vi "3010_2CAM.VI"() -> ()   [LabVIEW 2015]
uses:
  board.vis/Globals.vi
  <vilib>/Analysis/NI_AALBase.lvlib
panel:
  out "Signalverlaufgraph Cam 2":u16[](graph)=[28, 28, 29, 29, 30, 30, 31, 31, 32, 32, 33, 33, 34, 34, 35, 35, 36, 36, 37, 37, 38, 38, 39, 39, 40, 40, 41, 41, 42, 42, 43, 43, 44, 44, 45, 45, 46, 46, 47, 47, 48, 48, 49, 49, 50, 50, 51, 51, 52, 52, 53, 53, 54, 54, 55, 55, 56, 56, 57, 57, 58, 58, 59, 59, 60, 60, 61, 61, 62, 62, 63, 63, 64, 64, 65, 65, 66, 66, 67, 67, 68, 68, 69, 69, 70, 70, 71, 71, 72, 72, 73, 73, 74, 74, 75, 75, 76, 76, 77, 77, 78, 78, 79, 79, 80, 80, 81, 81, 82, 82, 83, 83, 84, 84, 85, 85, 86, 86, 87, 87, 88, 88, 89, 89, 90, 90, 91, 91, 92, 92, 93, 93, 94, 94, 95, 95, 96, 96, 97, 97, 98, 98, 99, 99, 100, 100, 101, 101, 102, 102, 103, 103, 104, 104, 105, 105, 106, 106, 107, 107, 108, 108, 109, 109, 110, 110, 111, 111, 112, 112, 113, 113, 114, 114, 115, 115, 116, 116, 117, 117, 118, 118, 119, 119, 120, 120, 121, 121, 122, 122, 123, 123, 124, 124, 125, 125, 126, 126, 127, 127, 128, 128, 129, 129, 130, 130, 131, 131, 132, 132, 133, 133, 134, 134, 135, 135, 136, 136, 137, 137, 138, 138, 139, 139, 140, 140, 141, 141, 142, 142, 143, 143, 144, 144, 145, 145, 146, 146, 147, 147, 148, 148, 149, 149, 150, 150, 151, 151, 152, 152, 153, 153, 154, 154, 155, 155, 156, 156, 157, 157, 158, 158, 159, 159, 160, 160, 161, 161, 162, 162, 163, 163, 164, 164, 165, 165, 166, 166, 167, 167, 168, 168, 169, 169, 170, 170, 171, 171, 172, 172, 173, 173, 174, 174, 175, 175, 176, 176, 177, 177, 178, 178, 179, 179, 180, 180, 181, 181, 182, 182, 183, 183, 184, 184, 185, 185, 186, 186, 187, 187, 188, 188, 189, 189, 190, 190, 191, 191, 192, 192, 193, 193, 194, 194, 195, 195, 196, 196, 197, 197, 198, 198, 199, 199, 200, 200, 201, 201, 202, 202, 203, 203, 204, 204, 205, 205, 206, 206, 207, 207, 208, 208, 209, 209, 210, 210, 211, 211, 212, 212, 213, 213, 214, 214, 215, 215, 216, 216, 217, 217, 218, 218, 219, 219, 220, 220, 221, 221, 222, 222, 223, 223, 224, 224, 225, 225, 226, 226, 227, 227, 228, 228, 229, 229, 230, 230, 231, 231, 232, 232, 233, 233, 234, 234, 235, 235, 236, 236, 237, 237, 238, 238, 239, 239, 240, 240, 241, 241, 242, 242, 243, 243, 244, 244, 245, 245, 246, 246, 247, 247, 248, 248, 249, 249, 250, 250, 251, 251, 252, 252, 253, 253, 254, 254, 255, 255, 256, 256, 257, 257, 258, 258, 259, 259, 260, 260, 261, 261, 262, 262, 263, 263, 264, 264, 265, 265, 266, 266, 267, 267, 268, 268, 269, 269, 270, 270, 271, 271, 272, 272, 273, 273, 274, 274, 275, 275, 276, 276, 277, 277, 278, 278, 279, 279, 280, 280, 281, 281, 282, 282, 283, 283, 284, 284, 285, 285, 286, 286, 287, 287, 288, 288, 289, 289, 290, 290, 291, 291, 292, 292, 293, 293, 294, 294, 295, 295, 296, 296, 297, 297, 298, 298, 299, 299, 300, 300, 301, 301, 302, 302, 303, 303, 304, 304, 305, 305, 306, 306, 307, 307, 308, 308, 309, 309, 310, 310, 311, 311, 312, 312, 313, 313, 314, 314, 315, 315, 316, 316, 317, 317, 318, 318, 319, 319, 320, 320, 321, 321, 322, 322, 323, 323, 324, 324, 325, 325, 326, 326, 327, 327, 328, 328, 329, 329, 330, 330, 331, 331, 332, 332, 333, 333, 334, 334, 335, 335, 336, 336, 337, 337, 338, 338, 339, 339, 340, 340, 341, 341, 342, 342, 343, 343, 344, 344, 345, 345, 346, 346, 347, 347, 348, 348, 349, 349, 350, 350, 351, 351, 352, 352, 353, 353, 354, 354, 355, 355, 356, 356, 357, 357, 358, 358, 359, 359, 360, 360, 361, 361, 362, 362, 363, 363, 364, 364, 365, 365, 366, 366, 367, 367, 368, 368, 369, 369, 370, 370, 371, 371, 372, 372, 373, 373, 374, 374, 375, 375, 376, 376, 377, 377, 378, 378, 379, 379, 380, 380, 381, 381, 382, 382, 383, 383, 384, 384, 385, 385, 386, 386, 387, 387, 388, 388, 389, 389, 390, 390, 391, 391, 392, 392, 393, 393, 394, 394, 395, 395, 396, 396, 397, 397, 398, 398, 399, 399, 400, 400, 401, 401, 402, 402, 403, 403, 404, 404, 405, 405, 406, 406, 407, 407, 408, 408, 409, 409, 410, 410, 411, 411, 412, 412, 413, 413, 414, 414, 415, 415, 416, 416, 417, 417, 418, 418, 419, 419, 420, 420, 421, 421, 422, 422, 423, 423, 424, 424, 425, 425, 426, 426, 427, 427, 428, 428, 429, 429, 430, 430, 431, 431, 432, 432, 433, 433, 434, 434, 435, 435, 436, 436, 437, 437, 438, 438, 439, 439, 440, 440, 441, 441, 442, 442, 443, 443, 444, 444, 445, 445, 446, 446, 447, 447, 448, 448, 449, 449, 450, 450, 451, 451, 452, 452, 453, 453, 454, 454, 455, 455, 456, 456, 457, 457, 458, 458, 459, 459, 460, 460, 461, 461, 462, 462, 463, 463, 464, 464, 465, 465, 466, 466, 467, 467, 468, 468, 469, 469, 470, 470, 471, 471, 472, 472, 473, 473, 474, 474, 475, 475, 476, 476, 477, 477, 478, 478, 479, 479, 480, 480, 481, 481, 482, 482, 483, 483, 484, 484, 485, 485, 486, 486, 487, 487, 488, 488, 489, 489, 490, 490, 491, 491, 492, 492, 493, 493, 494, 494, 495, 495, 496, 496, 497, 497, 498, 498, 499, 499, 500, 500, 501, 501, 502, 502, 503, 503, 504, 504, 505, 505, 506, 506, 507, 507, 508, 508, 509, 509, 510, 510, 511, 511, 512, 512, 513, 513, 514, 514, 515, 515, 516, 516, 517, 517, 518, 518, 519, 519, 520, 520, 521, 521, 522, 522, 523, 523, 524, 524, 525, 525, 526, 526, 527, 527, 528, 528, 529, 529, 530, 530, 531, 531, 532, 532, 533, 533, 534, 534, 535, 535, 536, 536, 537, 537, 538, 538, 539, 539, 540, 540, 541, 541, 542, 542, 543, 543, 544, 544, 544, 544, 544, 544, 544, 544, 544, 544, 544, 544, 544, 544, 544, 544, 544, 544, 544, 544, 544, 544, 544, 544, 544, 544, 544, 544, 544, 544, 544, 544, 544, 544, 544, 544, 544, 544, 544, 544, 544, 544, 544, 544, 544, 544, 544, 544, 544, 544, 544, 544, 544, 544, 544, 544]
  in  "extTrig":bool
  in  "ext. trig. slope":enum32{"1", "2", "3"}(radio)
  out "tRMS":dbl=8.272957184592048 format="%0#.1f"
  out "mean":dbl=3064.5285285285286 format="%#_4f"
  in  "rms_pixel":u16=100
  in  "is FFT":bool=TRUE
  in  "IR gain":bool
  in  "continuous":bool
  out "curr.block":u8=10
  out "Measure ON":bool
  in  "Board select\n1: board 1\n2: board 2\n3: both boards":u8=3
  in  "no.of blocks (nob)\npress enter":u32=1
  in  "block":u32(slide)=1 max=10 scale=0.9..1.0
  out "Signalverlaufgraph Board 2":u16[](graph)=[0, 0, 543, 543, 0, 1, 0, 0, 2, 2, 3, 3, 4, 4, 5, 5, 6, 6, 7, 7, 8, 8, 9, 9, 10, 10, 11, 11, 12, 12, 13, 13, 14, 14, 15, 15, 16, 16, 17, 17, 18, 18, 19, 19, 20, 20, 21, 21, 22, 22, 23, 23, 24, 24, 25, 25, 26, 26, 27, 27, 28, 28, 29, 29, 30, 30, 31, 31, 32, 32, 33, 33, 34, 34, 35, 35, 36, 36, 37, 37, 38, 38, 39, 39, 40, 40, 41, 41, 42, 42, 43, 43, 44, 44, 45, 45, 46, 46, 47, 47, 48, 48, 49, 49, 50, 50, 51, 51, 52, 52, 53, 53, 54, 54, 55, 55, 56, 56, 57, 57, 58, 58, 59, 59, 60, 60, 61, 61, 62, 62, 63, 63, 64, 64, 65, 65, 66, 66, 67, 67, 68, 68, 69, 69, 70, 70, 71, 71, 72, 72, 73, 73, 74, 74, 75, 75, 76, 76, 77, 77, 78, 78, 79, 79, 80, 80, 81, 81, 82, 82, 83, 83, 84, 84, 85, 85, 86, 86, 87, 87, 88, 88, 89, 89, 90, 90, 91, 91, 92, 92, 93, 93, 94, 94, 95, 95, 96, 96, 97, 97, 98, 98, 99, 99, 100, 100, 101, 101, 102, 102, 103, 103, 104, 104, 105, 105, 106, 106, 107, 107, 108, 108, 109, 109, 110, 110, 111, 111, 112, 112, 113, 113, 114, 114, 115, 115, 116, 116, 117, 117, 118, 118, 119, 119, 120, 120, 121, 121, 122, 122, 123, 123, 124, 124, 125, 125, 126, 126, 127, 127, 128, 128, 129, 129, 130, 130, 131, 131, 132, 132, 133, 133, 134, 134, 135, 135, 136, 136, 137, 137, 138, 138, 139, 139, 140, 140, 141, 141, 142, 142, 143, 143, 144, 144, 145, 145, 146, 146, 147, 147, 148, 148, 149, 149, 150, 150, 151, 151, 152, 152, 153, 153, 154, 154, 155, 155, 156, 156, 157, 157, 158, 158, 159, 159, 160, 160, 161, 161, 162, 162, 163, 163, 164, 164, 165, 165, 166, 166, 167, 167, 168, 168, 169, 169, 170, 170, 171, 171, 172, 172, 173, 173, 174, 174, 175, 175, 176, 176, 177, 177, 178, 178, 179, 179, 180, 180, 181, 181, 182, 182, 183, 183, 184, 184, 185, 185, 186, 186, 187, 187, 188, 188, 189, 189, 190, 190, 191, 191, 192, 192, 193, 193, 194, 194, 195, 195, 196, 196, 197, 197, 198, 198, 199, 199, 200, 200, 201, 201, 202, 202, 203, 203, 204, 204, 205, 205, 206, 206, 207, 207, 208, 208, 209, 209, 210, 210, 211, 211, 212, 212, 213, 213, 214, 214, 215, 215, 216, 216, 217, 217, 218, 218, 219, 219, 220, 220, 221, 221, 222, 222, 223, 223, 224, 224, 225, 225, 226, 226, 227, 227, 228, 228, 229, 229, 230, 230, 231, 231, 232, 232, 233, 233, 234, 234, 235, 235, 236, 236, 237, 237, 238, 238, 239, 239, 240, 240, 241, 241, 242, 242, 243, 243, 244, 244, 245, 245, 246, 246, 247, 247, 248, 248, 249, 249, 250, 250, 251, 251, 252, 252, 253, 253, 254, 254, 255, 255, 256, 256, 257, 257, 258, 258, 259, 259, 260, 260, 261, 261, 262, 262, 263, 263, 264, 264, 265, 265, 266, 266, 267, 267, 268, 268, 269, 269, 270, 270, 271, 271, 272, 272, 273, 273, 274, 274, 275, 275, 276, 276, 277, 277, 278, 278, 279, 279, 280, 280, 281, 281, 282, 282, 283, 283, 284, 284, 285, 285, 286, 286, 287, 287, 288, 288, 289, 289, 290, 290, 291, 291, 292, 292, 293, 293, 294, 294, 295, 295, 296, 296, 297, 297, 298, 298, 299, 299, 300, 300, 301, 301, 302, 302, 303, 303, 304, 304, 305, 305, 306, 306, 307, 307, 308, 308, 309, 309, 310, 310, 311, 311, 312, 312, 313, 313, 314, 314, 315, 315, 316, 316, 317, 317, 318, 318, 319, 319, 320, 320, 321, 321, 322, 322, 323, 323, 324, 324, 325, 325, 326, 326, 327, 327, 328, 328, 329, 329, 330, 330, 331, 331, 332, 332, 333, 333, 334, 334, 335, 335, 336, 336, 337, 337, 338, 338, 339, 339, 340, 340, 341, 341, 342, 342, 343, 343, 344, 344, 345, 345, 346, 346, 347, 347, 348, 348, 349, 349, 350, 350, 351, 351, 352, 352, 353, 353, 354, 354, 355, 355, 356, 356, 357, 357, 358, 358, 359, 359, 360, 360, 361, 361, 362, 362, 363, 363, 364, 364, 365, 365, 366, 366, 367, 367, 368, 368, 369, 369, 370, 370, 371, 371, 372, 372, 373, 373, 374, 374, 375, 375, 376, 376, 377, 377, 378, 378, 379, 379, 380, 380, 381, 381, 382, 382, 383, 383, 384, 384, 385, 385, 386, 386, 387, 387, 388, 388, 389, 389, 390, 390, 391, 391, 392, 392, 393, 393, 394, 394, 395, 395, 396, 396, 397, 397, 398, 398, 399, 399, 400, 400, 401, 401, 402, 402, 403, 403, 404, 404, 405, 405, 406, 406, 407, 407, 408, 408, 409, 409, 410, 410, 411, 411, 412, 412, 413, 413, 414, 414, 415, 415, 416, 416, 417, 417, 418, 418, 419, 419, 420, 420, 421, 421, 422, 422, 423, 423, 424, 424, 425, 425, 426, 426, 427, 427, 428, 428, 429, 429, 430, 430, 431, 431, 432, 432, 433, 433, 434, 434, 435, 435, 436, 436, 437, 437, 438, 438, 439, 439, 440, 440, 441, 441, 442, 442, 443, 443, 444, 444, 445, 445, 446, 446, 447, 447, 448, 448, 449, 449, 450, 450, 451, 451, 452, 452, 453, 453, 454, 454, 455, 455, 456, 456, 457, 457, 458, 458, 459, 459, 460, 460, 461, 461, 462, 462, 463, 463, 464, 464, 465, 465, 466, 466, 467, 467, 468, 468, 469, 469, 470, 470, 471, 471, 472, 472, 473, 473, 474, 474, 475, 475, 476, 476, 477, 477, 478, 478, 479, 479, 480, 480, 481, 481, 482, 482, 483, 483, 484, 484, 485, 485, 486, 486, 487, 487, 488, 488, 489, 489, 490, 490, 491, 491, 492, 492, 493, 493, 494, 494, 495, 495, 496, 496, 497, 497, 498, 498, 499, 499, 500, 500, 501, 501, 502, 502, 503, 503, 504, 504, 505, 505, 506, 506, 507, 507, 508, 508, 509, 509, 510, 510, 511, 511, 512, 512, 513, 513, 514, 514, 515, 515, 516, 516, 517, 517, 518, 518, 519, 519, 520, 520, 521, 521, 522, 522, 523, 523, 524, 524, 525, 525, 526, 526, 527, 527, 528, 528, 529, 529, 530, 530, 531, 531, 532, 532, 533, 533, 534, 534, 535, 535, 536, 536, 537, 537, 538, 538, 539, 539, 540, 540, 541, 541]
  out "Signalverlaufgraph":u16[](graph)=[544, 544, 545, 545, 49152, 1, 0, 148, 2, 2, 3, 3, 4, 4, 5, 5, 6, 6, 7, 7, 8, 8, 9, 9, 10, 10, 11, 11, 12, 12, 13, 13, 14, 14, 15, 15, 16, 16, 17, 17, 18, 18, 19, 19, 20, 20, 21, 21, 22, 22, 23, 23, 24, 24, 25, 25, 26, 26, 27, 27, 28, 28, 29, 29, 30, 30, 31, 31, 32, 32, 33, 33, 34, 34, 35, 35, 36, 36, 37, 37, 38, 38, 39, 39, 40, 40, 41, 41, 42, 42, 43, 43, 44, 44, 45, 45, 46, 46, 47, 47, 48, 48, 49, 49, 50, 50, 51, 51, 52, 52, 53, 53, 54, 54, 55, 55, 56, 56, 57, 57, 58, 58, 59, 59, 60, 60, 61, 61, 62, 62, 63, 63, 64, 64, 65, 65, 66, 66, 67, 67, 68, 68, 69, 69, 70, 70, 71, 71, 72, 72, 73, 73, 74, 74, 75, 75, 76, 76, 77, 77, 78, 78, 79, 79, 80, 80, 81, 81, 82, 82, 83, 83, 84, 84, 85, 85, 86, 86, 87, 87, 88, 88, 89, 89, 90, 90, 91, 91, 92, 92, 93, 93, 94, 94, 95, 95, 96, 96, 97, 97, 98, 98, 99, 99, 100, 100, 101, 101, 102, 102, 103, 103, 104, 104, 105, 105, 106, 106, 107, 107, 108, 108, 109, 109, 110, 110, 111, 111, 112, 112, 113, 113, 114, 114, 115, 115, 116, 116, 117, 117, 118, 118, 119, 119, 120, 120, 121, 121, 122, 122, 123, 123, 124, 124, 125, 125, 126, 126, 127, 127, 128, 128, 129, 129, 130, 130, 131, 131, 132, 132, 133, 133, 134, 134, 135, 135, 136, 136, 137, 137, 138, 138, 139, 139, 140, 140, 141, 141, 142, 142, 143, 143, 144, 144, 145, 145, 146, 146, 147, 147, 148, 148, 149, 149, 150, 150, 151, 151, 152, 152, 153, 153, 154, 154, 155, 155, 156, 156, 157, 157, 158, 158, 159, 159, 160, 160, 161, 161, 162, 162, 163, 163, 164, 164, 165, 165, 166, 166, 167, 167, 168, 168, 169, 169, 170, 170, 171, 171, 172, 172, 173, 173, 174, 174, 175, 175, 176, 176, 177, 177, 178, 178, 179, 179, 180, 180, 181, 181, 182, 182, 183, 183, 184, 184, 185, 185, 186, 186, 187, 187, 188, 188, 189, 189, 190, 190, 191, 191, 192, 192, 193, 193, 194, 194, 195, 195, 196, 196, 197, 197, 198, 198, 199, 199, 200, 200, 201, 201, 202, 202, 203, 203, 204, 204, 205, 205, 206, 206, 207, 207, 208, 208, 209, 209, 210, 210, 211, 211, 212, 212, 213, 213, 214, 214, 215, 215, 216, 216, 217, 217, 218, 218, 219, 219, 220, 220, 221, 221, 222, 222, 223, 223, 224, 224, 225, 225, 226, 226, 227, 227, 228, 228, 229, 229, 230, 230, 231, 231, 232, 232, 233, 233, 234, 234, 235, 235, 236, 236, 237, 237, 238, 238, 239, 239, 240, 240, 241, 241, 242, 242, 243, 243, 244, 244, 245, 245, 246, 246, 247, 247, 248, 248, 249, 249, 250, 250, 251, 251, 252, 252, 253, 253, 254, 254, 255, 255, 256, 256, 257, 257, 258, 258, 259, 259, 260, 260, 261, 261, 262, 262, 263, 263, 264, 264, 265, 265, 266, 266, 267, 267, 268, 268, 269, 269, 270, 270, 271, 271, 272, 272, 273, 273, 274, 274, 275, 275, 276, 276, 277, 277, 278, 278, 279, 279, 280, 280, 281, 281, 282, 282, 283, 283, 284, 284, 285, 285, 286, 286, 287, 287, 288, 288, 289, 289, 290, 290, 291, 291, 292, 292, 293, 293, 294, 294, 295, 295, 296, 296, 297, 297, 298, 298, 299, 299, 300, 300, 301, 301, 302, 302, 303, 303, 304, 304, 305, 305, 306, 306, 307, 307, 308, 308, 309, 309, 310, 310, 311, 311, 312, 312, 313, 313, 314, 314, 315, 315, 316, 316, 317, 317, 318, 318, 319, 319, 320, 320, 321, 321, 322, 322, 323, 323, 324, 324, 325, 325, 326, 326, 327, 327, 328, 328, 329, 329, 330, 330, 331, 331, 332, 332, 333, 333, 334, 334, 335, 335, 336, 336, 337, 337, 338, 338, 339, 339, 340, 340, 341, 341, 342, 342, 343, 343, 344, 344, 345, 345, 346, 346, 347, 347, 348, 348, 349, 349, 350, 350, 351, 351, 352, 352, 353, 353, 354, 354, 355, 355, 356, 356, 357, 357, 358, 358, 359, 359, 360, 360, 361, 361, 362, 362, 363, 363, 364, 364, 365, 365, 366, 366, 367, 367, 368, 368, 369, 369, 370, 370, 371, 371, 372, 372, 373, 373, 374, 374, 375, 375, 376, 376, 377, 377, 378, 378, 379, 379, 380, 380, 381, 381, 382, 382, 383, 383, 384, 384, 385, 385, 386, 386, 387, 387, 388, 388, 389, 389, 390, 390, 391, 391, 392, 392, 393, 393, 394, 394, 395, 395, 396, 396, 397, 397, 398, 398, 399, 399, 400, 400, 401, 401, 402, 402, 403, 403, 404, 404, 405, 405, 406, 406, 407, 407, 408, 408, 409, 409, 410, 410, 411, 411, 412, 412, 413, 413, 414, 414, 415, 415, 416, 416, 417, 417, 418, 418, 419, 419, 420, 420, 421, 421, 422, 422, 423, 423, 424, 424, 425, 425, 426, 426, 427, 427, 428, 428, 429, 429, 430, 430, 431, 431, 432, 432, 433, 433, 434, 434, 435, 435, 436, 436, 437, 437, 438, 438, 439, 439, 440, 440, 441, 441, 442, 442, 443, 443, 444, 444, 445, 445, 446, 446, 447, 447, 448, 448, 449, 449, 450, 450, 451, 451, 452, 452, 453, 453, 454, 454, 455, 455, 456, 456, 457, 457, 458, 458, 459, 459, 460, 460, 461, 461, 462, 462, 463, 463, 464, 464, 465, 465, 466, 466, 467, 467, 468, 468, 469, 469, 470, 470, 471, 471, 472, 472, 473, 473, 474, 474, 475, 475, 476, 476, 477, 477, 478, 478, 479, 479, 480, 480, 481, 481, 482, 482, 483, 483, 484, 484, 485, 485, 486, 486, 487, 487, 488, 488, 489, 489, 490, 490, 491, 491, 492, 492, 493, 493, 494, 494, 495, 495, 496, 496, 497, 497, 498, 498, 499, 499, 500, 500, 501, 501, 502, 502, 503, 503, 504, 504, 505, 505, 506, 506, 507, 507, 508, 508, 509, 509, 510, 510, 511, 511, 512, 512, 513, 513, 514, 514, 515, 515, 516, 516, 517, 517, 518, 518, 519, 519, 520, 520, 521, 521, 522, 522, 523, 523, 524, 524, 525, 525, 526, 526, 527, 527, 528, 528, 529, 529, 530, 530, 531, 531, 532, 532, 533, 533, 534, 534, 535, 535, 536, 536, 537, 537, 538, 538, 539, 539, 540, 540, 541, 541]
  out "boards recognised":u8=1
  in  "alloc mem":bool
  out "FREE \nRAM MB":dbl=14657.53515625
  out "BUILT-IN\nRAM MB":dbl=18096.171875
  out "SEC":dbl=1.0
  out "MB RAM":dbl=4.150390625
  in  "DAT in 10ns":u32
  in  "stop all":bool
  in  "start":bool
  in  "sample":u32(slide)=75 max=3000 scale=0.9..100.0
  in  "no.of samples (nos)":u32=100
  in  "exposuretime[ms]":dbl=1.0 format="%.3f"
  # "press Esc to stop measurement"
  # "exit here"
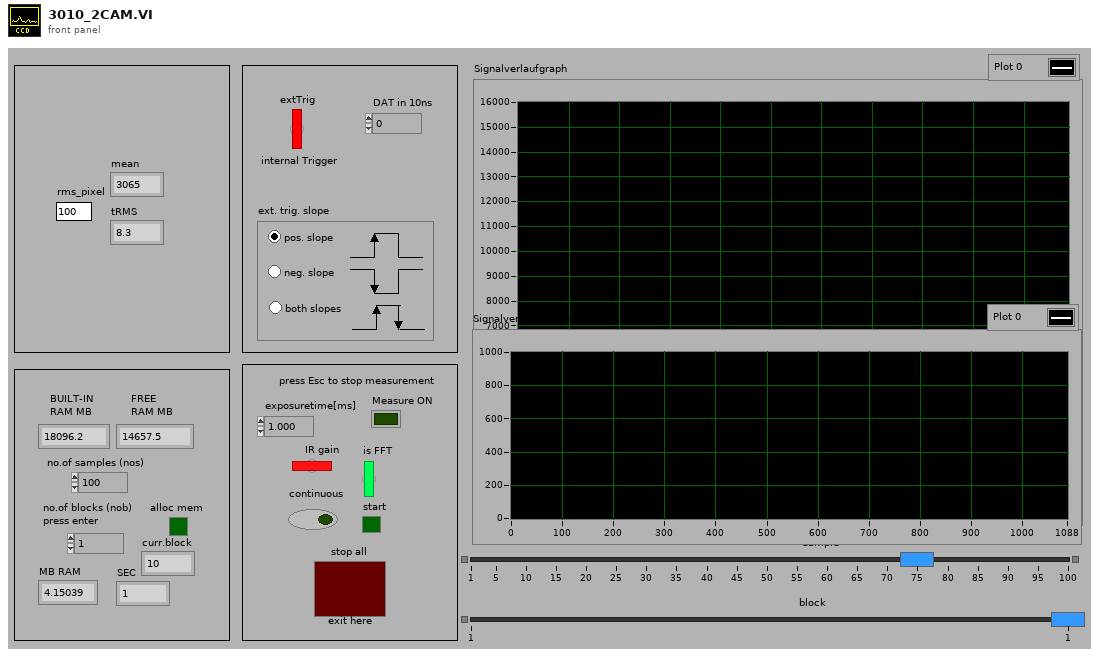
[diagram p1: front panel]
types:
  T1 = enum8{"Enabled", "Disabled", "Disabled and Grayed Out"}
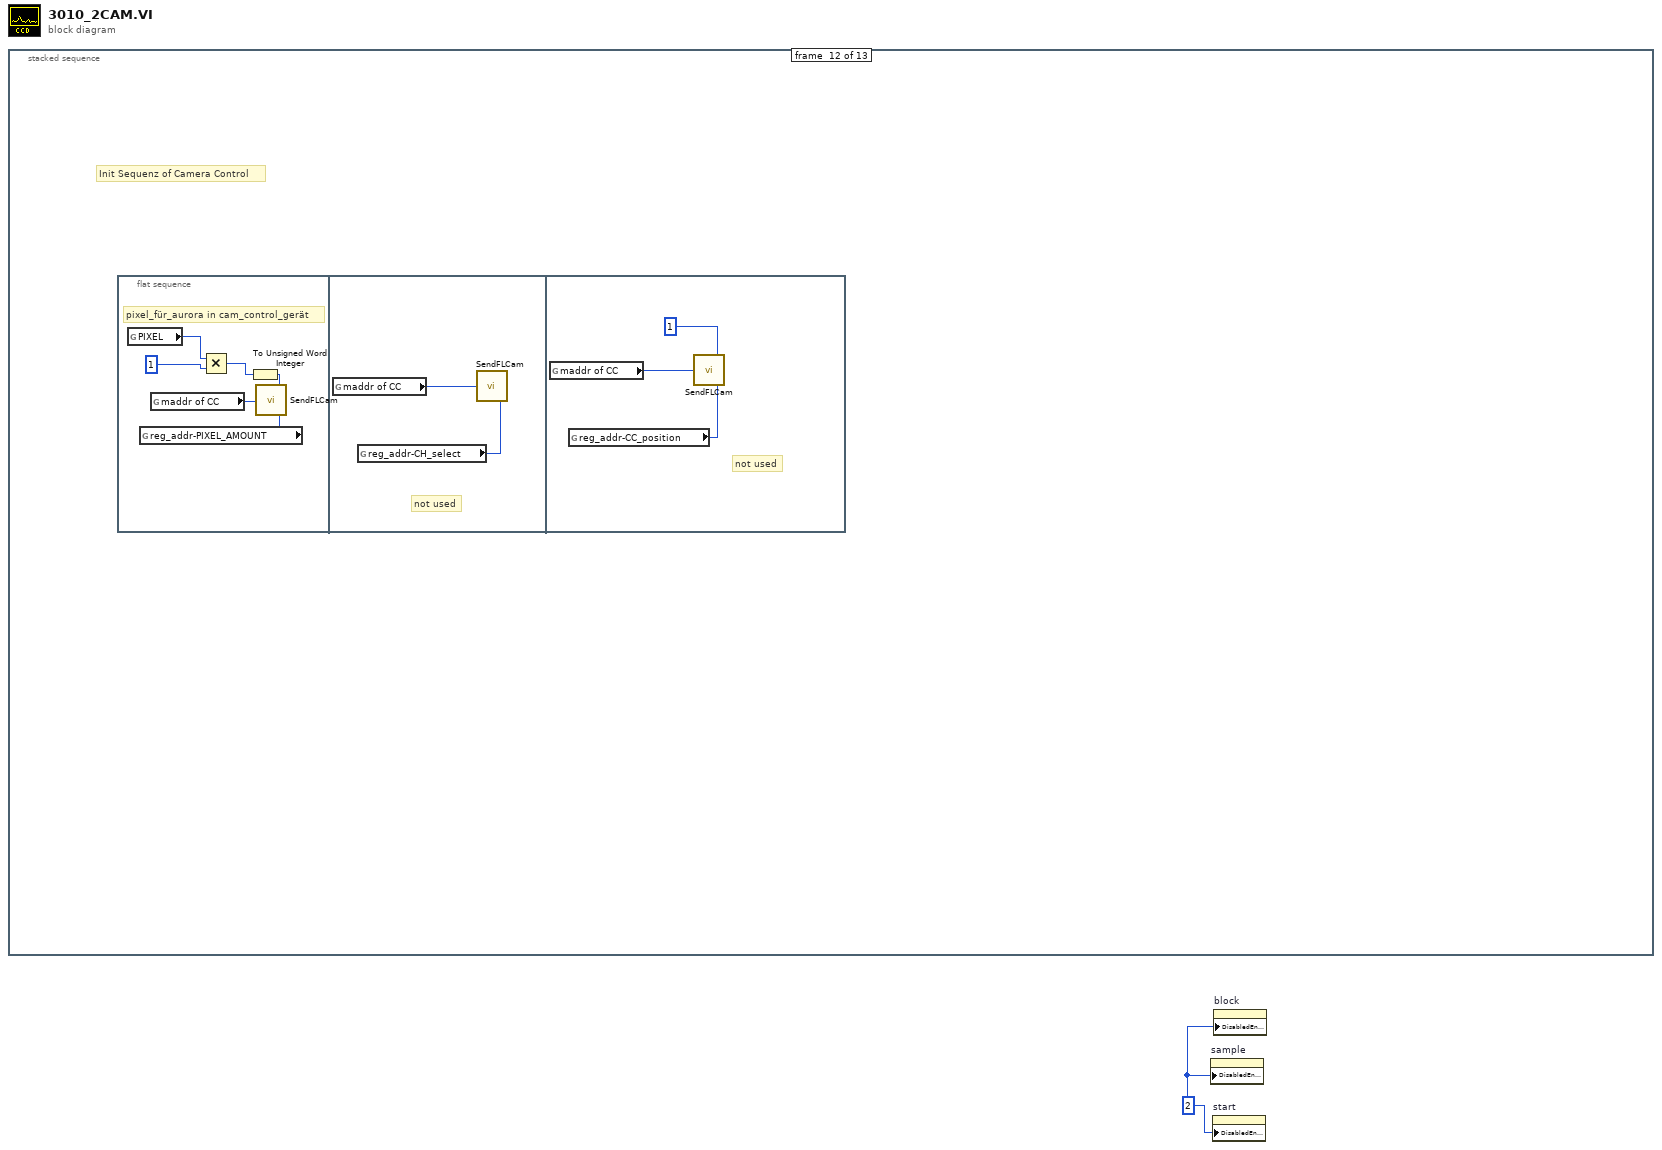
[diagram p0: block diagram]
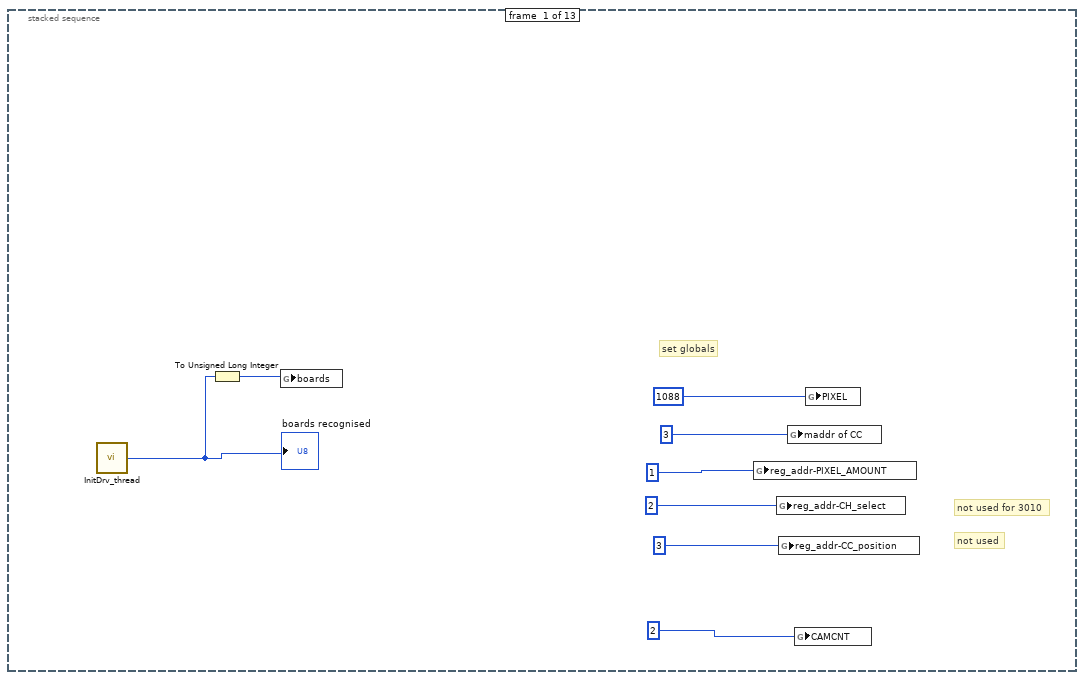
[diagram p2: hidden frame]
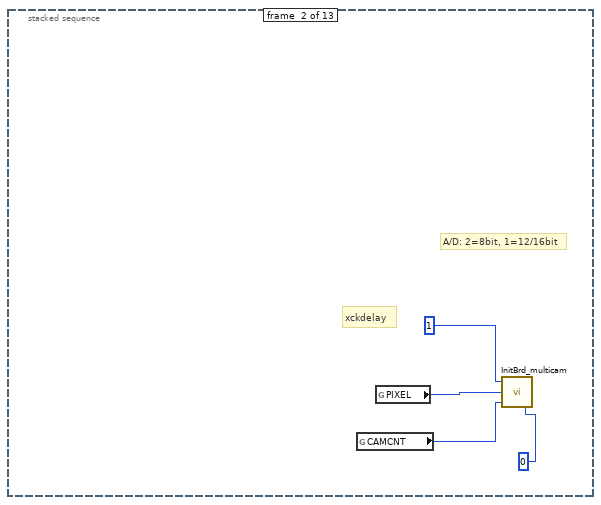
[diagram p3: hidden frame]
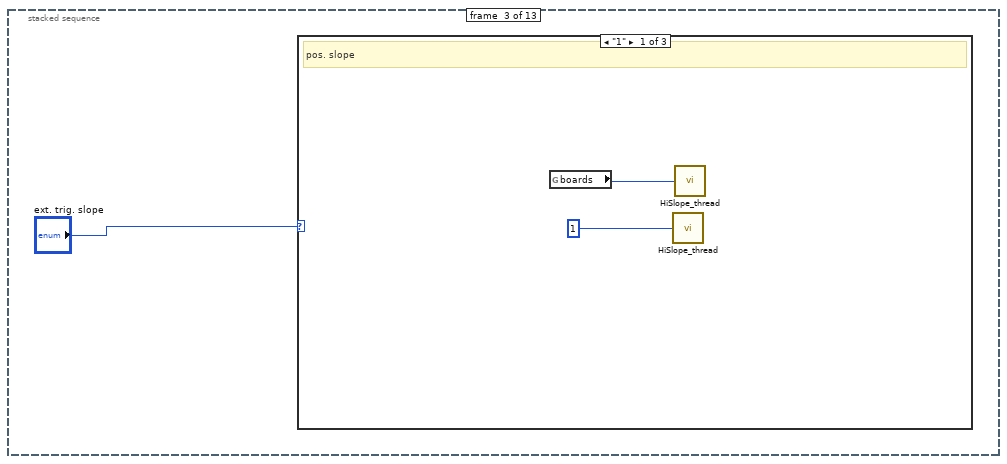
[diagram p4: hidden frame]
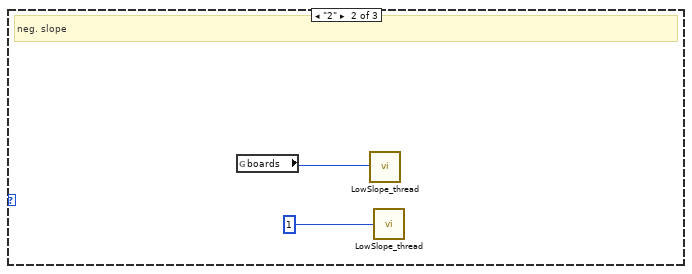
[diagram p5: hidden frame]
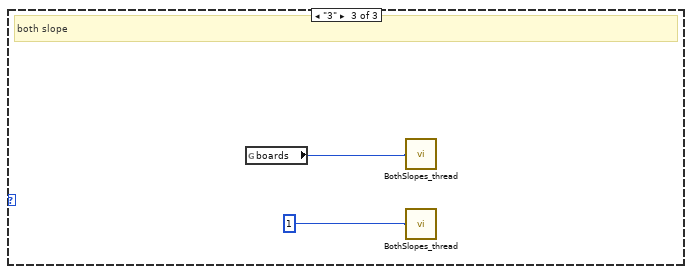
[diagram p6: hidden frame]
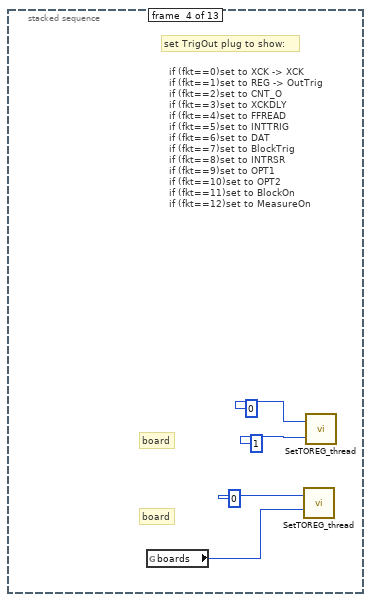
[diagram p7: hidden frame]
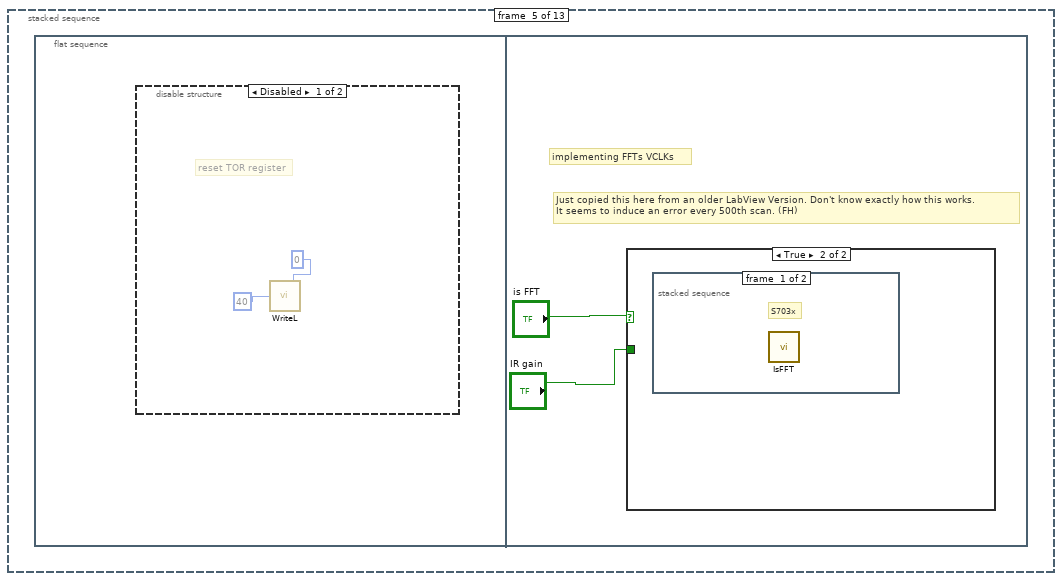
[diagram p8: hidden frame]
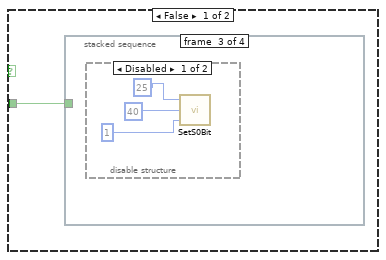
[diagram p10: hidden frame]
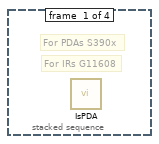
[diagram p11: hidden frame]
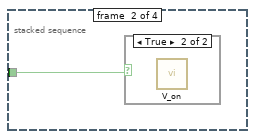
[diagram p12: hidden frame]
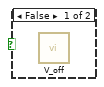
[diagram p13: hidden frame]
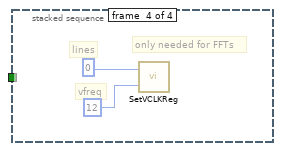
[diagram p15: hidden frame]
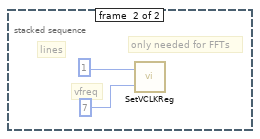
[diagram p16: hidden frame]
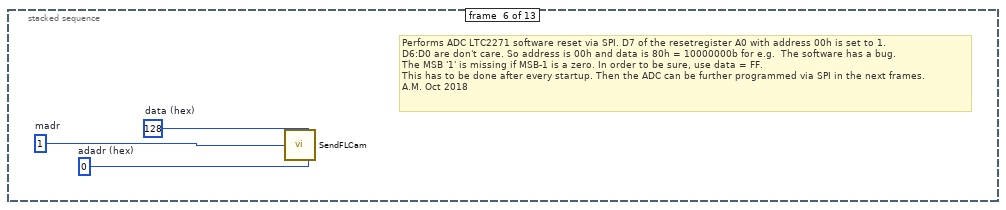
[diagram p17: hidden frame]
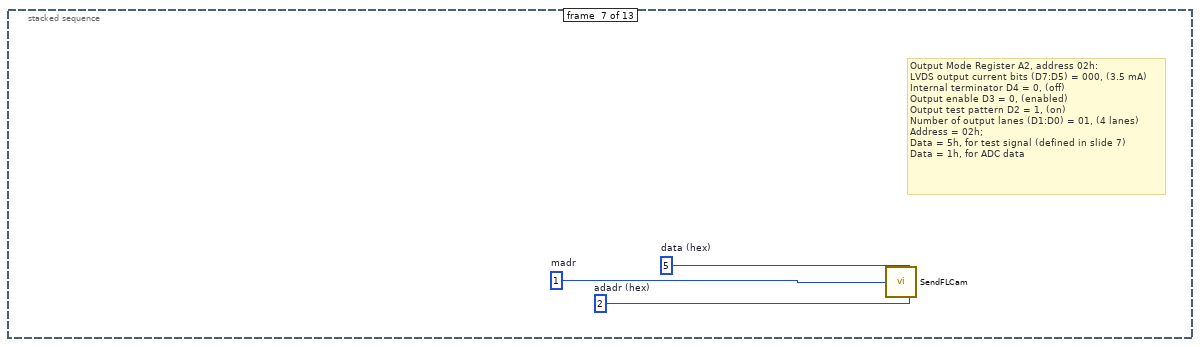
[diagram p18: hidden frame]
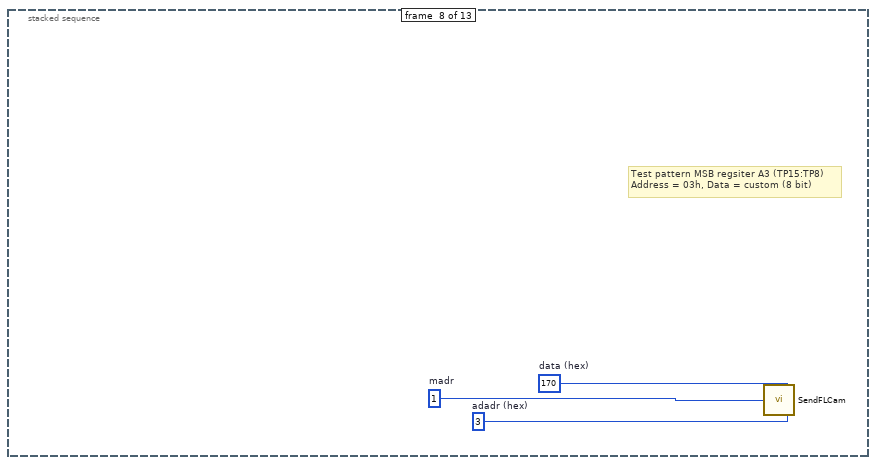
[diagram p19: hidden frame]
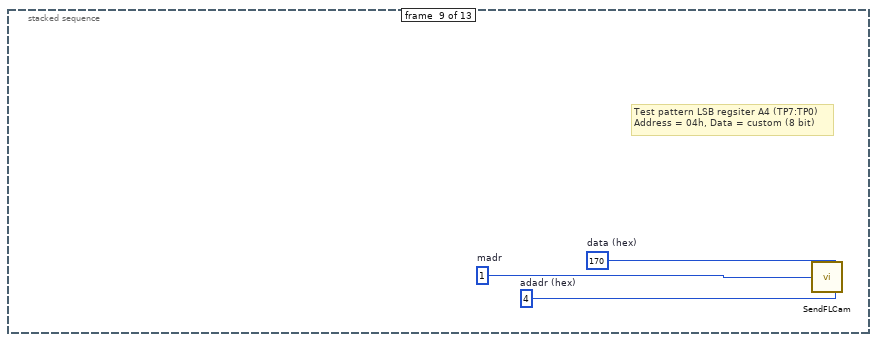
[diagram p20: hidden frame]
diagram:
  w1 = 2
  n1 = stacked-sequence {
    frame #0 {
      # "not used for 3010"
      # "not used"
      # "set globals"
      n2 = call "InitDrv_thread.vi"() -> ("Boards"=w7:u8)  [unwired: 1 in]
      "boards recognised" <- w7
      n3 = To Unsigned Long Integer(number=w7) -> (unsigned 32bit integer=w8:u32)
      n4 = global write "Globals.vi" "boards"(w8) -> ()
      n5 = global write "Globals.vi" "reg_addr-PIXEL_AMOUNT"(u8 1) -> ()
      n6 = global write "Globals.vi" "reg_addr-CH_select"(u8 2) -> ()
      n7 = global write "Globals.vi" "reg_addr-CC_position"(u8 3) -> ()
      n8 = global write "Globals.vi" "maddr of CC"(u8 3) -> ()
      n9 = global write "Globals.vi" "CAMCNT"(u32 2) -> ()
      n10 = global write "Globals.vi" "PIXEL"(u32 1088) -> ()
    }
    frame #1 {
      # "xckdelay"
      # "A/D: 2=8bit, 1=12/16bit"
      n11 = global read "Globals.vi" "CAMCNT"() -> (w10:u32)
      n12 = global read "Globals.vi" "PIXEL"() -> (w13:u32)
      n13 = call "InitBrd_multicam.vi"("xckdly"=u32 0, "camcnt"=w10, "pixel"=w13, "flag816"=u32 1) -> ()  [unwired: 2 in]
    }
    frame #2 {
      n14 = case shown="\"1\"" "ext. trig. slope" {
        frame "1" {
          # "pos. slope"
          n15 = global read "Globals.vi" "boards"() -> (w15:u32)
          n16 = call "HiSlope_thread.vi"("board"=u32 1) -> ()  [unwired: 1 in]
          n17 = call "HiSlope_thread.vi"("board"=w15) -> ()  [unwired: 1 in]
        }
        frame "2" {
          # "neg. slope"
          n18 = global read "Globals.vi" "boards"() -> (w18:u32)
          n19 = call "LowSlope_thread.vi"("board"=w18) -> ()  [unwired: 1 in]
          n20 = call "LowSlope_thread.vi"("board"=u32 1) -> ()  [unwired: 1 in]
        }
        frame "3" {
          # "both slope"
          n21 = global read "Globals.vi" "boards"() -> (w19:u32)
          n22 = call "BothSlopes_thread.vi"("board"=w19) -> ()  [unwired: 1 in]
          n23 = call "BothSlopes_thread.vi"("board"=u32 1) -> ()  [unwired: 1 in]
        }
      }
    }
    frame #3 {
      # "board"
      # "board"
      # "set TrigOut plug to show:"
      # "if (fkt==0)set to XCK -> XCK\nif (fkt==1)set to REG -> OutTrig\nif (fkt==2)set to CNT_O\nif (fkt==3)set to XCKDLY\nif (fkt==4)set to FFREAD\nif (fkt==5)set to INTTRIG\nif (fkt==6)set to DAT\nif (fkt==7)set to BlockTrig\nif (fkt==8)set to INTRSR\nif (fkt==9)set to OPT1\nif (fkt==10)set to OPT2\nif (fkt==11)set to BlockOn\nif (fkt==12)set to MeasureOn"
      n24 = global read "Globals.vi" "boards"() -> (w24:u32)
      n25 = call "SetTOREG_thread.vi"("board"=w24, "fkt"=u8 0) -> ()  [unwired: 1 in]
      n26 = call "SetTOREG_thread.vi"("board"=u32 1, "fkt"=u8 0) -> ()  [unwired: 1 in]
    }
    frame #4 {
      n27 = flat-sequence {
        frame #0 {
          n28 = disable-structure shown="Disabled" {
            frame Disabled {
              # "reset TOR register"
              n29 = call "WriteL.vi"("val"=u32 0, "offset"=u32 40) -> ()
            }
            frame Enabled {
            }
          }
        }
        frame #1 {
          # "implementing FFTs VCLKs"
          # "Just copied this here from an older LabView Version. Don't know exactly how this works.\nIt seems to induce an error every 500th scan. (FH)"
          n30 = case shown="True" "is FFT" {
            tunnel: "IR gain" -> [w29 _]
            frame False {
              n31 = stacked-sequence {
                tunnel: w29 -> [_ w30 _ _]
                frame #0 {
                  # "For IRs G11608"
                  # "For PDAs S390x"
                  n32 = call "IsPDA.vi"() -> ()  [unwired: 1 in]
                }
                frame #1 {
                  n33 = case shown="True" w30 {
                    frame False {
                      n34 = call "V_off.vi"() -> ()  [unwired: 1 in]
                    }
                    frame True {
                      n35 = call "V_on.vi"() -> ()  [unwired: 1 in]
                    }
                  }
                }
                frame #2 {
                  n36 = disable-structure shown="Disabled" {
                    frame Disabled {
                      n37 = call "SetS0Bit.vi"("drv"=u32 1, "Address"=u8 40, "bitnumber"=u32 25) -> ()
                    }
                    frame Enabled {
                    }
                  }
                }
                frame #3 {
                  # "only needed for FFTs"
                  # "vfreq"
                  # "lines"
                  n38 = call "SetVCLKReg.vi"("vfreq"=u8 12, "lines"=u32 0) -> ()  [unwired: 1 in]
                }
              }
            }
            frame True {
              n39 = stacked-sequence {
                frame #0 {
                  # "S703x"
                  n40 = call "IsFFT.vi"() -> ()  [unwired: 1 in]
                }
                frame #1 {
                  # "only needed for FFTs"
                  # "vfreq"
                  # "lines"
                  n41 = call "SetVCLKReg.vi"("vfreq"=u8 7, "lines"=u32 1) -> ()  [unwired: 1 in]
                }
              }
            }
          }
        }
      }
    }
    frame #5 {
      w38 = u16 128  # data (hex)
      w39 = u8 0  # adadr (hex)
      w40 = u8 1  # madr
      # "Performs ADC LTC2271 software reset via SPI. D7 of the resetregister A0 with address 00h is set to 1.\nD6:D0 are don't care. So address is 00h and data is 80h = 10000000b for e.g.  The software has a bug.\nThe MSB '1' is missing if MSB-1 is a zero. In order to be sure, use data = FF.\nThis has to be done after every startup. Then the ADC can be further programmed via SPI in the next frames.\nA.M. Oct 2018"
      n42 = call "SendFLCam.vi"("madr"=w40, "data"=w38, "adadr"=w39) -> ()
    }
    frame #6 {
      w41 = u16 5  # data (hex)
      w42 = u8 2  # adadr (hex)
      w43 = u8 1  # madr
      # "Output Mode Register A2, address 02h:\nLVDS output current bits (D7:D5) = 000, (3.5 mA)\nInternal terminator D4 = 0, (off)\nOutput enable D3 = 0, (enabled)\nOutput test pattern D2 = 1, (on)\nNumber of output lanes (D1:D0) = 01, (4 lanes)\nAddress = 02h;\nData = 5h, for test signal (defined in slide 7)\nData = 1h, for ADC data"
      n43 = call "SendFLCam.vi"("madr"=w43, "data"=w41, "adadr"=w42) -> ()
    }
    frame #7 {
      w44 = u16 170  # data (hex)
      w45 = u8 3  # adadr (hex)
      w46 = u8 1  # madr
      # "Test pattern MSB regsiter A3 (TP15:TP8)\nAddress = 03h, Data = custom (8 bit)"
      n44 = call "SendFLCam.vi"("madr"=w46, "data"=w44, "adadr"=w45) -> ()
    }
    frame #8 {
      w47 = u16 170  # data (hex)
      w48 = u8 4  # adadr (hex)
      w49 = u8 1  # madr
      # "Test pattern LSB regsiter A4 (TP7:TP0)\nAddress = 04h, Data = custom (8 bit)"
      n45 = call "SendFLCam.vi"("madr"=w49, "data"=w47, "adadr"=w48) -> ()
    }
    frame #9 {
      # "bit31 must be set for enabling DAT(add 0x80000000) to REG 0x20"
      # "is only valid for external trigger!"
      # "this examples shows how to set the DAT (delay after trigger)"
      n46 = Equal To 0?(x="DAT in 10ns") -> (x = 0?=w51:bool)
      n47 = case shown="True" w51 {
        tunnel: "DAT in 10ns" -> [w56 _]
        frame False {
          w53 = u32 32
          n48 = global read "Globals.vi" "boards"() -> (w55:u32)
          n49 = Add(x=u32 2147483648, y=w56) -> (x+y=w54:u32)
          n50 = call "WriteL_thread.vi"("val"=w54, "board"=w55, "offset"=w53) -> ()
          n51 = call "WriteL_thread.vi"("val"=w54, "board"=u32 1, "offset"=w53) -> ()
        }
        frame True {
          n52 = global read "Globals.vi" "boards"() -> (w62:u32)
          n53 = call "WriteL_thread.vi"("val"=u32 0, "board"=u32 1, "offset"=u32 32) -> ()
          n54 = call "WriteL_thread.vi"("val"=u32 0, "board"=w62, "offset"=u32 32) -> ()
        }
      }
    }
    frame #10 {
      w66 = FALSE
      w71 = 2
      # "set gain must be last in init sequence"
      n55 = global read "Globals.vi" "boards"() -> (w65:u32)
      n56 = case shown="1, Default" w65 {
        frame 2 {
          w79 = TRUE
          n57 = property on="Signalverlaufgraph" class="WFGraph (strict)"("Height"=u8 170) -> ()  [unwired: 2 in, 2 out]
          n58 = global write "Globals.vi" "board_sel"(u8 3) -> ()
          n59 = property on="boards recognised" class="DigNum (strict)"("Visible"=w79) -> ()  [unwired: 2 in, 2 out]
          n60 = property on="Board select\n1: board 1\n2: board 2\n3: both boards" class="DigNum (strict)"("Visible"=w79) -> ()  [unwired: 2 in, 2 out]
          n61 = property on="Signalverlaufgraph Board 2" class="WFGraph (strict)"("Visible"=w79) -> ()  [unwired: 2 in, 2 out]
        }
        frame 1, Default {
          w80 = FALSE
          n62 = global write "Globals.vi" "board_sel"(u8 1) -> ()
          n63 = property on="Signalverlaufgraph" class="WFGraph (strict)"("Height"=400) -> ()  [unwired: 2 in, 2 out]
          n64 = property on="Board select\n1: board 1\n2: board 2\n3: both boards" class="DigNum (strict)"("Visible"=w80) -> ()  [unwired: 2 in, 2 out]
          n65 = property on="Signalverlaufgraph Board 2" class="WFGraph (strict)"("Visible"=w80) -> ()  [unwired: 2 in, 2 out]
          n66 = property on="boards recognised" class="DigNum (strict)"("Visible"=w80) -> ()  [unwired: 2 in, 2 out]
        }
      }
      n67 = call "SetAdGain_thread.vi"("gain"=u8 0, "board"=u32 1) -> ()  [unwired: 1 in]
      n68 = call "SetAdGain_thread.vi"("gain"=u8 0, "board"=w65) -> ()  [unwired: 1 in]
      n69 = property on="sample" class="Slide (strict)"("DisabledEnum"=w71) -> ()  [unwired: 2 in, 2 out]
      n70 = property on="continuous" class="Bool (strict)"("DisabledEnum"=w71) -> ()  [unwired: 2 in, 2 out]
      n71 = property on="start" class="Bool (strict)"("DisabledEnum"=w71) -> ()  [unwired: 2 in, 2 out]
      n72 = property on="stop all" class="Bool (strict)"("DisabledEnum"=0) -> ()  [unwired: 2 in, 2 out]
      n73 = property on="block" class="Slide (strict)"("DisabledEnum"=w71) -> ()  [unwired: 2 in, 2 out]
      n74 = global read "Globals.vi" "CAMCNT"() -> (w64:u32)
      n75 = case shown="2" w64 {
        frame 2 {
          n76 = global write "Globals.vi" "board_sel"(u8 3) -> ()
          n77 = property on="Signalverlaufgraph" class="WFGraph (strict)"("Height"=u8 170) -> ()  [unwired: 2 in, 2 out]
          n78 = property on="Signalverlaufgraph Cam 2" class="WFGraph (strict)"("Visible"=TRUE) -> ()  [unwired: 2 in, 2 out]
        }
        frame 1, Default {
          n79 = property on="Signalverlaufgraph" class="WFGraph (strict)"("Height"=400) -> ()  [unwired: 2 in, 2 out]
          n80 = property on="Signalverlaufgraph Cam 2" class="WFGraph (strict)"("Visible"=FALSE) -> ()  [unwired: 2 in, 2 out]
        }
      }
      n81 = property on="continuous" class="Bool (strict)"("Value"=w66) -> ()  [unwired: 2 in, 2 out]
      n82 = property on="Measure ON" class="Bool (strict)"("Value"=w66) -> ()  [unwired: 2 in, 2 out]
    }
    frame #11 {
      # "Init Sequenz of Camera Control"
      n83 = flat-sequence {
        frame #0 {
          # "pixel_für_aurora in cam_control_gerät"
          n84 = global read "Globals.vi" "PIXEL"() -> (w84:u32)
          n85 = global read "Globals.vi" "reg_addr-PIXEL_AMOUNT"() -> (w88:u8)
          n86 = global read "Globals.vi" "maddr of CC"() -> (w87:u8)
          n87 = Multiply(x=w84, y=1) -> (x*y=w85:u32)
          n88 = To Unsigned Word Integer(number=w85) -> (unsigned 16bit integer=w86:u16)
          n89 = call "SendFLCam.vi"("madr"=w87, "data"=w86, "adadr"=w88) -> ()
        }
        frame #1 {
          # "not used"
          n90 = global read "Globals.vi" "maddr of CC"() -> (w90:u8)
          n91 = global read "Globals.vi" "reg_addr-CH_select"() -> (w89:u8)
          n92 = call "SendFLCam.vi"("madr"=w90, "adadr"=w89) -> ()  [unwired: 1 in]
        }
        frame #2 {
          # "not used"
          n93 = global read "Globals.vi" "maddr of CC"() -> (w93:u8)
          n94 = global read "Globals.vi" "reg_addr-CC_position"() -> (w92:u8)
          n95 = call "SendFLCam.vi"("madr"=w93, "data"=u16 1, "adadr"=w92) -> ()
        }
      }
    }
    frame #12 {
      n96 = while {
        stop <- w95 stop-if-true
        n97 = event shown="[0] Timeout" {
          selector: _ -> [_ _ _ _ _ _ _ _ _ _]
          dyn-events: _ -> [_ _ _ _ _ _ _ _ _ _]
          timeout: 100 -> [_ _ _ _ _ _ _ _ _ _]
          tunnel: [_ _ _ _ _ _ _ _ w223 _] -> w95
          event Timeout {
            # "only refresh the frames if measure on"
            # "compares measure on signal from hardware with measure on lamp\nwhen diffrent than write new measure on value to lamp"
            # "timout excecutes every 100ms"
            # "userinfo of RAM, MeasureOB, Curr.Block and setting display event in cont mode"
            n98 = event-data() -> ()  [unwired: 1 in, 3 out]
            n99 = call "ReadB.vi"("Offset"=u32 64) -> ("Data"=w112:u8)
            n100 = call "FreeMemInfo.vi"() -> ("PhysicalSpace"=→"BUILT-IN\nRAM MB":dbl, "PhysicalFreeSpace"=→"FREE \nRAM MB":dbl)  [unwired: 1 in]
            n101 = Number To Boolean Array(number=w112) -> (Boolean array=w111:bool[])
            n102 = property on="Measure ON" class="Bool (strict)"() -> ("Value"=w106:bool)  [unwired: 2 in, 2 out]
            n103 = Index Array(array=w111, index=5) -> (element=w102:bool)
            n104 = Not Equal?(x=w106, y=w102) -> (x != y?=w105:bool)
            n105 = case shown="True" w105 {
              tunnel: w102 -> [_ w116]
              frame False {
              }
              frame True {
                n106 = property on="Measure ON" class="Bool (strict)"("Val(Sgnl)"=w116) -> ()  [unwired: 2 in, 2 out]
              }
            }
            n107 = property on="continuous" class="Bool (strict)"() -> ("DisabledEnum"=w99:T1)  [unwired: 2 in, 2 out]
            n108 = property on="continuous" class="Bool (strict)"() -> ("Value"=w108:bool)  [unwired: 2 in, 2 out]
            n109 = To Unsigned Byte Integer(number=w99) -> (unsigned 8bit integer=w100:u8)
            n110 = Equal?(x=w100, y=u8 0) -> (x = y?=w107:bool)
            n111 = And(x=w108, y=w107) -> (x .and. y?=w104:bool)
            n112 = And(x=w104, y=w102) -> (x .and. y?=w103:bool)
            n113 = call "ReadB.vi"("Offset"=u32 88) -> ("Data"=w97:u8)
            n114 = global read "Globals.vi" "CAMCNT"() -> (w96:u32)
            n115 = case shown="True" w103 {
              frame False {
              }
              frame True {
                # "refresh RMS.\nMaybe this is not a good style.\nIt's not clear to me which values are \nincluded to RMS measurement.\nBetter would be a refresh when all\nblocks are done."
                # "trigger the \ndisplay event"
                n116 = property on="rms_pixel" class="DigNum (strict)"() -> ("Value"=w117:u16)  [unwired: 2 in, 2 out]
                n117 = property on="sample" class="Slide (strict)"() -> ("Value"=w118:u32)  [unwired: 2 in, 2 out]
                n118 = property on="sample" class="Slide (strict)"("Val(Sgnl)"=w118) -> ()  [unwired: 2 in, 2 out]
                n119 = property on="rms_pixel" class="DigNum (strict)"("Val(Sgnl)"=w117) -> ()  [unwired: 2 in, 2 out]
              }
            }
            n120 = Divide(x=w97, y=w96) -> (x/y=→"curr.block":dbl)
          }
          event "Measure ON": Value Change {
            # "triggers on value change of measure on. this happens on start of measurement and after measurement\nwhen continuous: not after finishing all blocks, only when exiting measurement"
            n121 = event-data() -> ("NewVal"=w119:bool)  [unwired: 1 in, 5 out]
            n122 = property on="continuous" class="Bool (strict)"() -> ("Value"=w120:bool)  [unwired: 2 in, 2 out]
            n123 = And(x=w120, y=w119) -> (x .and. y?=w121:bool)
            n124 = case shown="False" w119 {
              frame False {
                n125 = property on="stop all" class="Bool (strict)"("DisabledEnum"=0) -> ()  [unwired: 2 in, 2 out]
              }
              frame True {
              }
            }
            n126 = case shown="True" w121 {
              frame False {
              }
              frame True {
                n127 = property on="stop all" class="Bool (strict)"("DisabledEnum"=2) -> ()  [unwired: 2 in, 2 out]
              }
            }
          }
          event "Board select\n1: board 1\n2: board 2\n3: both boards": Value Change {
            # "selecting number of cams"
            n128 = event-data() -> ()  [unwired: 1 in, 6 out]
            n129 = global read "Globals.vi" "boards"() -> (w124:u32)
            n130 = case shown="2" w124 {
              frame 0, Default {
              }
              frame 2 {
                n131 = global write "Globals.vi" "board_sel"("Board select\n1: board 1\n2: board 2\n3: both boards") -> ()
              }
            }
          }
          event "continuous": Value Change {
            # "setting continuos mode"
            n132 = event-data() -> ()  [unwired: 1 in, 6 out]
            n133 = case shown="False" "continuous" {
              tunnel: [u8 0 u8 1] -> w126
              frame False {
              }
              frame True {
              }
            }
            n134 = call "contFFLoop.vi"("Numeric"=w126) -> ()  [unwired: 1 in]
          }
          event "alloc mem": Value Change {
            w136 = 0
            # "update params"
            # "Setup DMA"
            n135 = event-data() -> ()  [unwired: 1 in, 6 out]
            n136 = global read "Globals.vi" "cams_amount"() -> (w133:u8)
            n137 = global read "Globals.vi" "nob"() -> (w134:u32)
            n138 = global read "Globals.vi" "nos"() -> (w135:u32)
            n139 = To Unsigned Long Integer(number=w133) -> (unsigned 32bit integer=w132:u32)
            n140 = global read "Globals.vi" "boards"() -> (w139:u32)
            n141 = Multiply(x=w132, y=w134) -> (x*y=w130:u32)
            n142 = Multiply(x=w132, y=w135) -> (x*y=w131:u32)
            n143 = case shown="2" w139 {
              selector: w139 -> [_ w140]
              tunnel: w131 -> [_ w141]
              tunnel: w130 -> [_ w142]
              frame 1, Default {
              }
              frame 2 {
                # "Setup DMA"
                n144 = call "SetupDMA_thread.vi"("blocks"=w142, "nos"=w141, "Drv"=w140) -> ()  [unwired: 2 in]
              }
            }
            n145 = call "SetupDMA_thread.vi"("blocks"=w130, "nos"=w131, "Drv"=u32 1) -> ()  [unwired: 2 in]
            n146 = property on="continuous" class="Bool (strict)"("DisabledEnum"=w136) -> ()  [unwired: 2 in, 2 out]
            n147 = property on="block" class="Slide (strict)"("DisabledEnum"=w136) -> ()  [unwired: 2 in, 2 out]
            n148 = property on="sample" class="Slide (strict)"("DisabledEnum"=w136) -> ()  [unwired: 2 in, 2 out]
            n149 = property on="exposuretime[ms]" class="DigNum (strict)"() -> ("Value"=w138:dbl)  [unwired: 2 in, 2 out]
            n150 = property on="start" class="Bool (strict)"("DisabledEnum"=w136) -> ()  [unwired: 2 in, 2 out]
            n151 = property on="exposuretime[ms]" class="DigNum (strict)"("Val(Sgnl)"=w138) -> ()  [unwired: 2 in, 2 out]
          }
          event "start": Mouse Down {
            # "start measurement"
            # "only 1st PCI board is used for ext. trig."
            # "ext. block trig\n0: internal: Space\n1: PCI \"I\"\n2: S1\n3: S2"
            # "block trigger 0/1\n0: internal -> next block is started immediately \n1: external -> each block has an own trigger"
            n152 = event-data() -> ()  [unwired: 1 in, 8 out]
            n153 = global read "Globals.vi" "exp time"() -> (w149:dbl)
            n154 = Multiply(x=1000.0, y=w149) -> (x*y=w151:dbl)
            n155 = global read "Globals.vi" "board_sel"() -> (w145:u8)
            n156 = To Unsigned Long Integer(number=w151) -> (unsigned 32bit integer=w147:u32)
            n157 = case shown="True" "extTrig" {
              tunnel: [u8 0 u8 1] -> w144
              frame False {
              }
              frame True {
              }
            }
            n158 = call "ReadFFLoop_thread.vi"("blocktrigger"=u8 0, "btrig_ch"=u8 0, "ExtTrig"=w144, "cam_sel"=w145, "exptus"=w147) -> ()  [unwired: 1 in]
          }
          event "sample", "block": Value Change {
            w170 = u32 1
            # "when selecting a value\nbigger than possible\nnos or nob, a dummy \nvalue \"1\" is chosen\n\nTODO:\ninsert error handling\nwith lower values than 1"
            # "display"
            n159 = event-data() -> ()  [unwired: 1 in, 6 out]
            n160 = global read "Globals.vi" "boards"() -> (w171:u32)
            n161 = global read "Globals.vi" "nob"() -> (w162:u32)
            n162 = global read "Globals.vi" "nos"() -> (w169:u32)
            n163 = Greater Or Equal?(x=w162, y="block") -> (x >= y?=w165:bool)
            n164 = Greater Or Equal?(x=w169, y="sample") -> (x >= y?=w168:bool)
            n165 = case shown="True" w165 {
              tunnel: [u32 1 w186] -> w164
              tunnel: "block" -> [_ w186]
              frame False {
                n166 = call "Display Message to User"() -> ()  [unwired: 10 in, 2 out]
              }
              frame True {
              }
            }
            n167 = case shown="False" w168 {
              tunnel: [u32 1 w188] -> w167
              tunnel: "sample" -> [_ w188]
              frame False {
                n168 = call "Display Message to User2"() -> ()  [unwired: 10 in, 2 out]
              }
              frame True {
              }
            }
            n169 = global read "Globals.vi" "CAMCNT"() -> (w155:u32)
            n170 = global read "Globals.vi" "PIXEL"() -> (w159:u32)
            n171 = Subtract(x=w167, y=w170) -> (x-y=w156:u32)
            n172 = Subtract(x=w164, y=w170) -> (x-y=w157:u32)
            n173 = case shown="2" w171 {
              selector: w171 -> [_ w193]
              tunnel: w156 -> [_ w194]
              tunnel: w157 -> [_ w191]
              frame 0, Default {
              }
              frame 2 {
                n174 = global read "Globals.vi" "PIXEL"() -> (w189:u32)
                n175 = To Long Integer(number=w189) -> (32bit integer=w190:i32)
                n176 = Initialize Array(u16 100, w190) -> (w196:u16[])
                n177 = call "ReturnFrame.vi"("Data Values In"=w196, "curr_nob"=w191, "curr_nos"=w194, "Drv"=w193) -> ("Data Values Out"=→"Signalverlaufgraph Board 2":u16[])  [unwired: 1 in]
              }
            }
            n178 = To Long Integer(number=w159) -> (32bit integer=w160:i32)
            n179 = Initialize Array(u16 100, w160) -> (w174:u16[])
            n180 = Multiply(x=w155, y=w156) -> (x*y=w154:u32)
            n181 = call "ReturnFrame.vi"("Data Values In"=w174, "curr_nob"=w157, "curr_nos"=w154, "Drv"=u32 1) -> ("Data Values Out"=→"Signalverlaufgraph":u16[])  [unwired: 1 in]
            n182 = global read "Globals.vi" "CAMCNT"() -> (w158:u32)
            n183 = case shown="2" w158 {
              tunnel: w157 -> [_ w178]
              tunnel: w154 -> [_ w176]
              frame 1, Default {
              }
              frame 2 {
                n184 = Add(x=w176, y=u32 1) -> (x+y=w177:u32)
                n185 = global read "Globals.vi" "PIXEL"() -> (w183:u32)
                n186 = To Long Integer(number=w183) -> (32bit integer=w182:i32)
                n187 = Initialize Array(u16 100, w182) -> (w179:u16[])
                n188 = call "ReturnFrame.vi"("Data Values In"=w179, "curr_nob"=w178, "curr_nos"=w177, "Drv"=u32 1) -> ("Data Values Out"=→"Signalverlaufgraph Cam 2":u16[])  [unwired: 1 in]
              }
            }
          }
          event "no.of samples (nos)", "no.of blocks (nob)\npress enter", "exposuretime[ms]": Value Change {
            # "calculation of MB RAM an SEC and setting scale max"
            # "MB"
            # "ushort"
            n189 = event-data() -> ()  [unwired: 1 in, 7 out]
            n190 = global read "Globals.vi" "PIXEL"() -> (w222:u32)
            n191 = Multiply(x="no.of samples (nos)", y=w222) -> (x*y=w220:u32)
            n192 = Multiply(x=w220, y=u32 2) -> (x*y=w200:u32)
            n193 = global read "Globals.vi" "boards"() -> (w221:u32)
            n194 = global read "Globals.vi" "cams_amount"() -> (w199:u8)
            n195 = global read "Globals.vi" "nos"() -> (w204:u32)
            n196 = global read "Globals.vi" "nob"() -> (w202:u32)
            n197 = To Unsigned Long Integer(number=w199) -> (unsigned 32bit integer=w198:u32)
            n198 = Multiply(x=w198, y=w200) -> (x*y=w197:u32)
            n199 = Multiply(x=w197, y=w221) -> (x*y=w210:u32)
            n200 = To Double Precision Float(number=w210) -> (double precision float=w209:dbl)
            n201 = To Double Precision Float(number=w204) -> (double precision float=w203:dbl)
            n202 = Divide(x=w209, y=1048576.0) -> (x/y=w212:dbl)
            n203 = To Double Precision Float(number=w202) -> (double precision float=w201:dbl)
            n204 = To Double Precision Float(number="no.of blocks (nob)\npress enter") -> (double precision float=w207:dbl)
            n205 = property on="sample" class="Slide (strict)"("Scale.Maximum"=w203) -> ()  [unwired: 2 in, 2 out]
            n206 = property on="block" class="Slide (strict)"("Scale.Maximum"=w201) -> ()  [unwired: 2 in, 2 out]
            n207 = Multiply(x=w212, y=w207) -> (x*y=→"MB RAM":dbl)
            n208 = global write "Globals.vi" "nos"("no.of samples (nos)") -> ()
            n209 = Multiply(x="no.of samples (nos)", y="no.of blocks (nob)\npress enter") -> (x*y=w205:u32)
            n210 = global write "Globals.vi" "nob"("no.of blocks (nob)\npress enter") -> ()
            n211 = To Double Precision Float(number=w205) -> (double precision float=w206:dbl)
            n212 = global write "Globals.vi" "exp time"("exposuretime[ms]") -> ()
            n213 = Multiply(x="exposuretime[ms]", y=w206) -> (x*y=w218:dbl)
            n214 = Divide(x=w218, y=1000.0) -> (x/y=→"SEC":dbl)
          }
          event "stop all": Value Change {
            # "exit"
            n215 = event-data() -> ()  [unwired: 1 in, 6 out]
            n216 = stacked-sequence {
              tunnel: [_ TRUE] -> w223
              frame #0 {
                n217 = call "FFStop.vi"() -> ()  [unwired: 1 in]
              }
              frame #1 {
                # "do not omit, or next call of driver will go wrong."
                n218 = call "Exit.vi"() -> ()  [unwired: 1 in]
              }
            }
          }
          event "rms_pixel": Value Change {
            # "one array with all values (except first 10)\nat index Pixel from all blocks"
            n219 = event-data() -> ()  [unwired: 1 in, 6 out]
            n220 = global read "Globals.vi" "nos"() -> (w229:u32)
            n221 = global read "Globals.vi" "nob"() -> (w230:u32)
            n222 = for {
              N: w230 -> [_]
              tunnel: w229 -> [w231]
              tunnel: [w233] -> w226 mode=concatenating
              i -> [w237]
              # "delete first 10 values"
              # "array of all values\nat index Pixel"
              n223 = To Long Integer(number=w231) -> (32bit integer=w232:i32)
              n224 = for {
                N: w232 -> [_]
                tunnel: w237 -> [w242]
                tunnel: [w246] -> w234 mode=indexing
                i -> [w244]
                # "use only value at index \"Pixel\""
                # "init array of size PIXEL\nwith value 100"
                n225 = global read "Globals.vi" "PIXEL"() -> (w238:u32)
                n226 = To Long Integer(number=w238) -> (32bit integer=w239:i32)
                n227 = To Unsigned Long Integer(number=w242) -> (unsigned 32bit integer=w243:u32)
                n228 = To Unsigned Long Integer(number=w244) -> (unsigned 32bit integer=w245:u32)
                n229 = Initialize Array(u16 100, w239) -> (w248:u16[])
                n230 = call "ReturnFrame.vi"("Data Values In"=w248, "curr_nob"=w243, "curr_nos"=w245, "Drv"=u32 1) -> ("Data Values Out"=w247:u16[])  [unwired: 1 in]
                n231 = To Long Integer(number="rms_pixel") -> (32bit integer=w240:i32)
                n232 = Index Array(array=w247, index=w240) -> (element=w246:u16)
              }
              n233 = Delete From Array(array=w234, length=10, index=0) -> (array with subset deleted=w233:u16[])  [unwired: 1 out]
            }
            n234 = To Double Precision Float(number=w226) -> (double precision float=w225:dbl[])
            n235 = call <vilib>:"Std Deviation and Variance.vi"("X"=w225) -> ("mean"=→"mean":dbl, "standard deviation"=→"tRMS":dbl)  [unwired: 1 in, 1 out]
          }
        }
      }
    }
  }
  n236 = property on="sample" class="Slide (strict)"("DisabledEnum"=w1) -> ()  [unwired: 2 in, 2 out]
  n237 = property on="start" class="Bool (strict)"("DisabledEnum"=w1) -> ()  [unwired: 2 in, 2 out]
  n238 = property on="block" class="Slide (strict)"("DisabledEnum"=w1) -> ()  [unwired: 2 in, 2 out]
